vi "Point Shoot Cloud Grid.vi"(8 "Error in (no error)":errorcluster, 9 "Y":dbl=3.1847341119828343e-07 format="%#_6p", 10 "X":dbl=-2.397470098003396e-07 format="%#_6p", 11 "Method":enum16{"init", "run", "end"}(ring)=enum."run") -> (0 "Error out":errorcluster)   [LabVIEW 2014]
doc: "Example of a measurement VI to be used in the \"Point & Shoot\" tool in Follow Me mode as external VI.\n\nThis example performs multiple bias spectroscopy measurements after each movement.\n\n- Nanonis Programming Interface -"
uses:
  <userlib>/Nanonis Prog Interface V5/Nanonis Prog Interface.lvlib
panel:
  in  "Experiment Name":string
  in  "Num Point":i32
  out "Y (m)":sgl
  out "X (m)":sgl
  in  "pattern file":path
  in  "start":string="start"
  in  "Color":u32(colorbox)=14680303
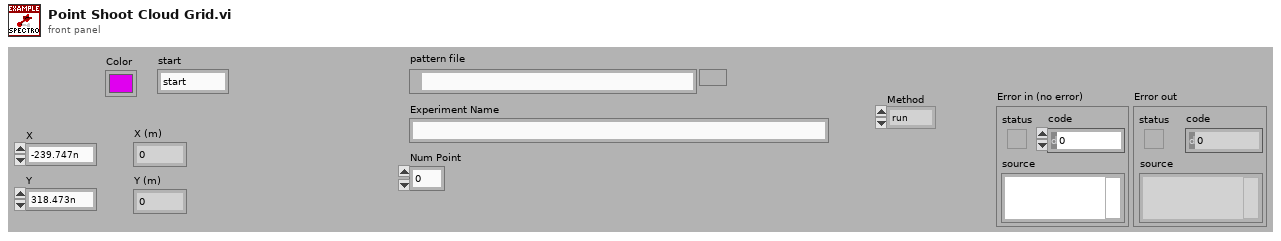
[diagram p1: front panel]
types:
  T1 = cluster{"X (m)":sgl, "Y (m)":sgl, "Text":string, "Color":u32, "Visible":bool}[]
  T2 = cluster{"X (m)":sgl, "Y (m)":sgl, "Text":string, "Color":u32, "Visible":bool}
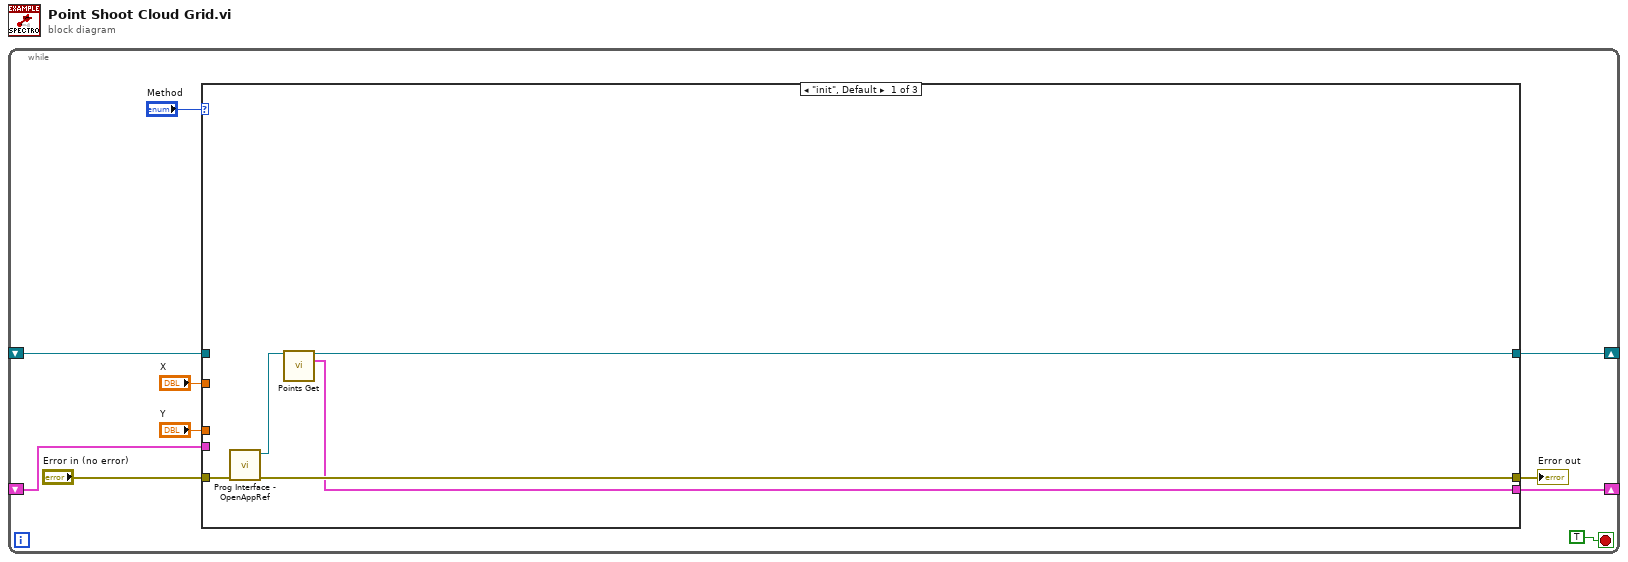
[diagram p0: block diagram]
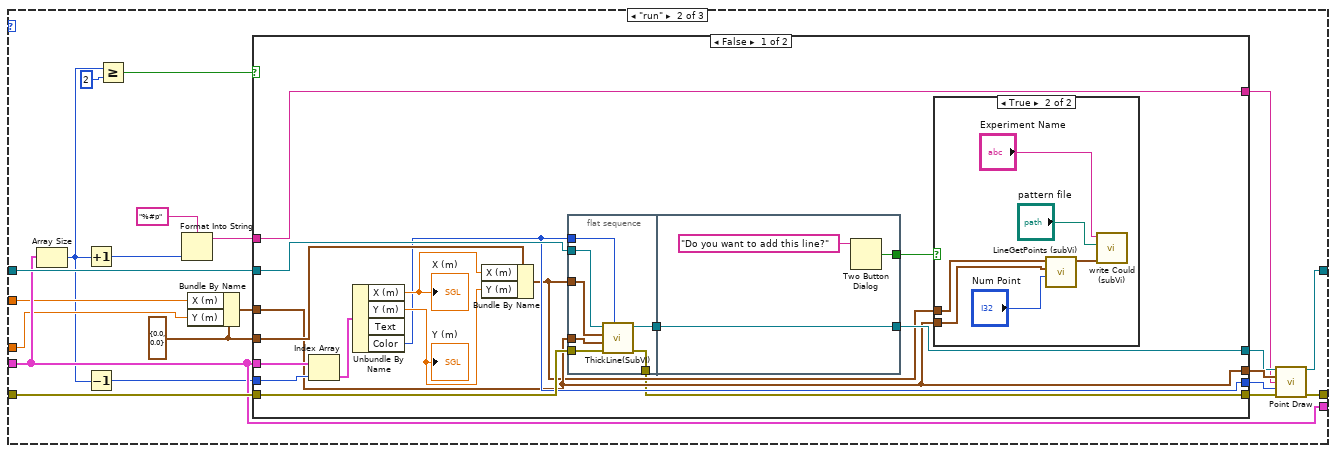
[diagram p2: hidden frame]
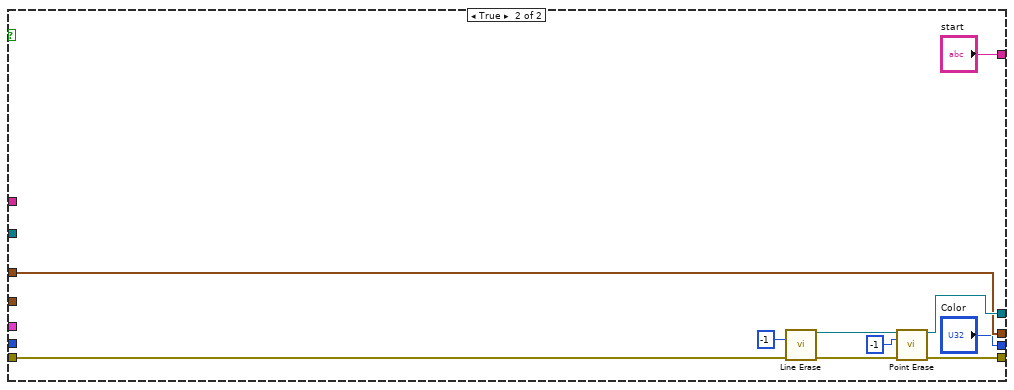
[diagram p4: hidden frame]
diagram:
  n1 = while {
    shift-right: [w4] -> _
    shift-left: _ -> [w3]
    shift-right: [w2] -> _
    shift-left: _ -> [w1]
    stop <- TRUE stop-if-true
    n2 = case shown="\"init\", Default" "Method" {
      tunnel: "Error in (no error)" -> [w15 w34 w81]
      tunnel: [w14 w33 w81] -> w7
      tunnel: "X" -> [_ w30 _]
      tunnel: "Y" -> [_ w31 _]
      tunnel: [w11 w36 w80] -> w4
      tunnel: w3 -> [_ w35 w80]
      tunnel: [w12 w32 w79] -> w2
      tunnel: w1 -> [_ w32 w79]
      frame "init", Default {
        n3 = call <userlib>:"Prog Interface - OpenAppRef.vi"("Error in (no error)"=w15) -> ("Error out"=w14:errorcluster, "Application reference"=w13:refnum<vi>)  [unwired: 5 in]
        n4 = call <userlib>:"Points Get.vi"("Application ref in"=w13) -> ("Application ref out"=w11:refnum<vi>, "Points"=w12:T1)  [unwired: 12 in, 1 out]
      }
      frame "run" {
        w24 = cluster{"X (m)":sgl, "Y (m)":sgl} {"X (m)"=0.0, "Y (m)"=0.0} ("End Point Coordinates")
        n5 = Array Size(array=w32) -> (size(s)=w19:i32)
        n6 = Increment(x=w19) -> (x+1=w17:i32)
        n7 = Decrement(x=w19) -> (x-1=w29:i32)
        n8 = Greater Or Equal?(x=w19, y=2) -> (x >= y?=w18:bool)
        n9 = Format Into String(format string="%#p", w17) -> (resulting string=w22:string)  [unwired: 2 in, 1 out]
        n10 = Bundle By Name(cluster=w24, "X (m)"=w30, "Y (m)"=w31) -> (w23:cluster{"X (m)":sgl, "Y (m)":sgl})
        n11 = case shown="False" w18 {
          tunnel: w32 -> [w52 _]
          tunnel: w29 -> [w51 _]
          tunnel: [w41 w72] -> w28
          tunnel: w35 -> [w47 _]
          tunnel: [w46 w74] -> w27
          tunnel: w34 -> [w45 w73]
          tunnel: [w38 w69] -> w26
          tunnel: w24 -> [w44 _]
          tunnel: w23 -> [w41 w72]
          tunnel: w22 -> [w42 _]
          tunnel: [w42 "start"] -> w21
          tunnel: [w43 "Color"] -> w20
          frame False {
            n12 = Index Array(array=w52, index=w51) -> (element=w50:T2)
            n13 = Unbundle By Name(w50) -> ("X (m)"=w49:sgl, "Y (m)"=w48:sgl, "Color"=w43:u32)  [unwired: 1 out]
            "X (m)" <- w49
            "Y (m)" <- w48
            n14 = Bundle By Name(cluster=w44, "X (m)"=w49, "Y (m)"=w48) -> (w40:cluster{"X (m)":sgl, "Y (m)":sgl})
            n15 = flat-sequence {
              tunnel: w47 -> [w59]
              tunnel: w45 -> [w57]
              tunnel: w43 -> [w56]
              tunnel: w41 -> [w55]
              tunnel: w40 -> [w54]
              tunnel: [w58] -> w39
              tunnel: [w53] -> w38
              tunnel: [w62] -> w46
              tunnel: w39 -> [w62]
              tunnel: [w60] -> w37
              frame #0 {
                n16 = call "ThickLine(SubVI).vi"("Color"=w56, "error in (no error)"=w57, "End Point Coordinates"=w55, "End Point Coordinates 2"=w54, "Application in"=w59) -> ("error out"=w53:errorcluster, "Application out"=w58:refnum<vi>)  [unwired: 5 in]
              }
              frame #1 {
                n17 = Two Button Dialog(message="Do you want to add this line?") -> (T button?=w60:bool)  [unwired: 2 in]
              }
            }
            n18 = case shown="True" w37 {
              tunnel: w41 -> [_ w68]
              tunnel: w40 -> [_ w67]
              frame False {
              }
              frame True {
                n19 = call "LineGetPoints (subVi).vi"("Num Point"="Num Point", "End Point Coordinates"=w68, "Start Point Coordinates"=w67) -> ("Array"=w65:cluster{"X (m)":sgl, "Y (m)":sgl}[])  [unwired: 8 in]
                n20 = call "write Could (subVi).vi"("Array"=w65, "Experiment"="pattern file", "Experiment Name"="Experiment Name") -> ()  [unwired: 9 in]
              }
            }
          }
          frame True {
            n21 = call <userlib>:"Line Erase.vi"("Line index (-1=All lines)"=-1, "error in (no error)"=w73) -> ("Application ref out"=w78:refnum<vi>, "error out"=w77:errorcluster)  [unwired: 12 in]
            n22 = call <userlib>:"Point Erase.vi"("Application ref in"=w78, "Point index (-1=All points)"=-1, "error in (no error)"=w77) -> ("Application ref out"=w74:refnum<vi>, "error out"=w69:errorcluster)  [unwired: 11 in]
          }
        }
        n23 = call <userlib>:"Point Draw.vi"("Application ref in"=w27, "Point Coordinates"=w28, "Text"=w21, "Color"=w20, "error in (no error)"=w26) -> ("Application ref out"=w36:refnum<vi>, "error out"=w33:errorcluster)  [unwired: 9 in]
      }
      frame "end" {
      }
    }
    "Error out" <- w7
  }
